vi "SwapNodes.vi"(9 "Node2":refnum<data-value>, 11 "Node1":refnum<data-value>) -> ()   [LabVIEW 2010]
uses:
  Node.ctl
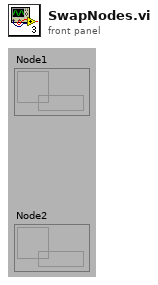
[diagram p1: front panel]
types:
  T1 = typedef "Node.ctl" = cluster{"Name":string, "Next":variant, "Previous":variant}
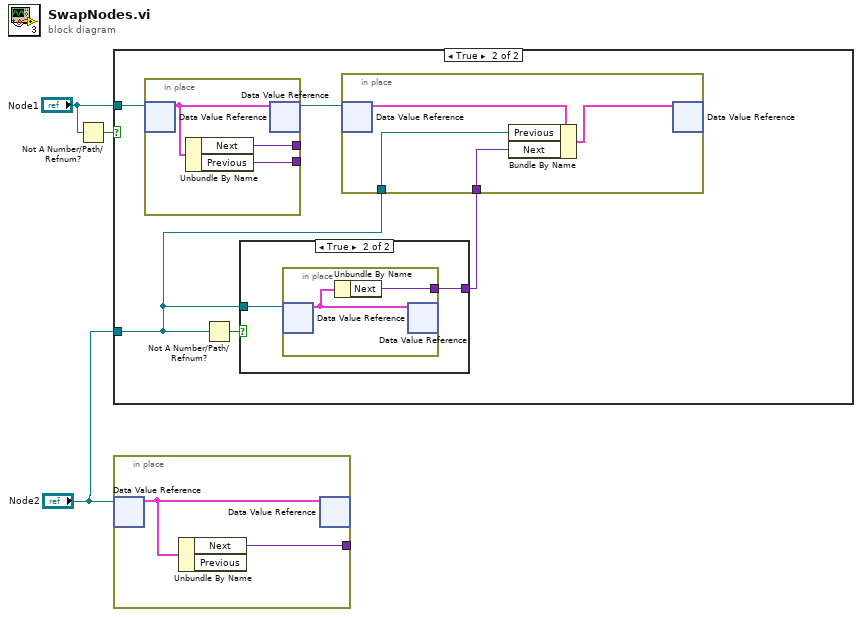
[diagram p0: block diagram]
diagram:
  n1 = Not A Number/Path/Refnum?(number/path/refnum="Node1") -> (NaN/Path/Refnum?=w2:bool)
  n2 = case shown="True" w2 {
    tunnel: "Node1" -> [_ w8]
    tunnel: "Node2" -> [_ w5]
    frame False {
    }
    frame True {
      n3 = in-place {
        in-place-border: [w19] -> _
        in-place-border: [w17] -> _
        n4 = in-place-dvr #1(w8) -> (w18:T1)  [unwired: 1 out]
        n5 = Unbundle By Name(w18) -> ("Next"=w19:variant, "Previous"=w17:variant)
        n6 = in-place-dvr #1(w18) -> (w7:refnum<data-value>)  [unwired: 1 out]
      }
      n7 = Not A Number/Path/Refnum?(number/path/refnum=w5) -> (NaN/Path/Refnum?=w6:bool)
      n8 = case shown="True" w6 {
        tunnel: w5 -> [_ w10]
        tunnel: [_ w9] -> w4
        frame False {
        }
        frame True {
          n9 = in-place {
            in-place-border: [w11] -> w9
            n10 = in-place-dvr #2(w10) -> (w12:T1)  [unwired: 1 out]
            n11 = Unbundle By Name(w12) -> ("Next"=w11:variant)
            n12 = in-place-dvr #2(w12) -> ()  [unwired: 2 out]
          }
        }
      }
      n13 = in-place {
        in-place-border: w5 -> [w15]
        in-place-border: w4 -> [w13]
        n14 = in-place-dvr #3(w7) -> (w16:T1)  [unwired: 1 out]
        n15 = Bundle By Name(cluster=w16, "Previous"=w15, "Next"=w13) -> (w14:T1)
        n16 = in-place-dvr #3(w14) -> ()  [unwired: 2 out]
      }
    }
  }
  n17 = in-place {
    in-place-border: [w21] -> _
    n18 = in-place-dvr #4("Node2") -> (w20:T1)  [unwired: 1 out]
    n19 = Unbundle By Name(w20) -> ("Next"=w21:variant)  [unwired: 1 out]
    n20 = in-place-dvr #4(w20) -> ()  [unwired: 2 out]
  }
